vi "SnapImage.vi"(6 "timeout in ms (1000)":i32=1000, 8 "error in (no error)":errorcluster, 11 "Camera":refnum<class "Camera.lvclass">) -> (0 "error out":errorcluster, 2 "buffer":i32=-1, 3 "Camera out":refnum<class "Camera.lvclass">)   [LabVIEW 2015, in "Camera.lvclass"]
doc: "---------------------------------------------------------------\nJKI State Machine Objects™\nhttp://jki.net/state-machine-objects/\nCopyright (C) 2005-2015, JKI <info@jki.net>\nALL RIGHTS RESERVEDJKI State Machine Objects (SMO) 1.0.0.4\nJKI - JKI\nCopyright (c) 2015, JKI"
uses:
  Camera.lvclass
  Camera.lvclass/Camera.ctl
panel:
  # "For instructions on how to use the JKI State Machine Objects, examples and video tutorials, visit:\nhttp://jki.net/state-machine-objects/\n\nJKI State Machine Objects™\nhttp://jki.net/state-machine-objects/\nCopyright (C) 2005-2015, JKI <info@jki.net>\nALL RIGHTS RESERVED"
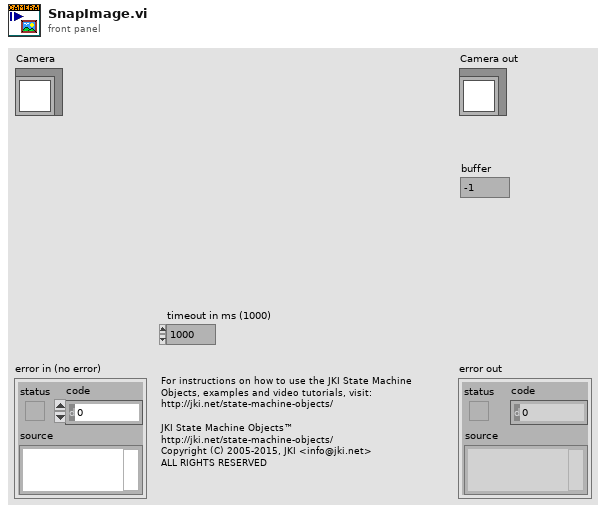
[diagram p1: front panel]
types:
  T1 = typedef "Camera.lvclass/PrivateData--Ref.ctl" = refnum<data-value>
  T2 = typedef "Camera.lvclass/PrivateData--Cluster.ctl" = cluster{"Public Events":T3, "Protected Events":T4, "Private Events":T5, "Dependencies":T6}
  T3 = typedef "Camera.lvclass/PublicEvents--Cluster.ctl" = cluster{"NewImage":refnum<user-event>, "ImageSaved":refnum<user-event>}
  T4 = typedef "Camera.lvclass/ProtectedEvents--Cluster.ctl" = cluster{"placeholder":refnum<user-event>}
  T5 = typedef "Camera.lvclass/PrivateEvents--Cluster.ctl" = cluster{"Snap Image":refnum<user-event>, "Save Image":refnum<user-event>, "Get Image":refnum<user-event>}
  T6 = typedef "Camera.Simulated.lvclass/Dependencies--Cluster.ctl" = cluster{"CircularBuffer.ImageData":refnum<class "CircularBuffer.ImageData.lvclass">}
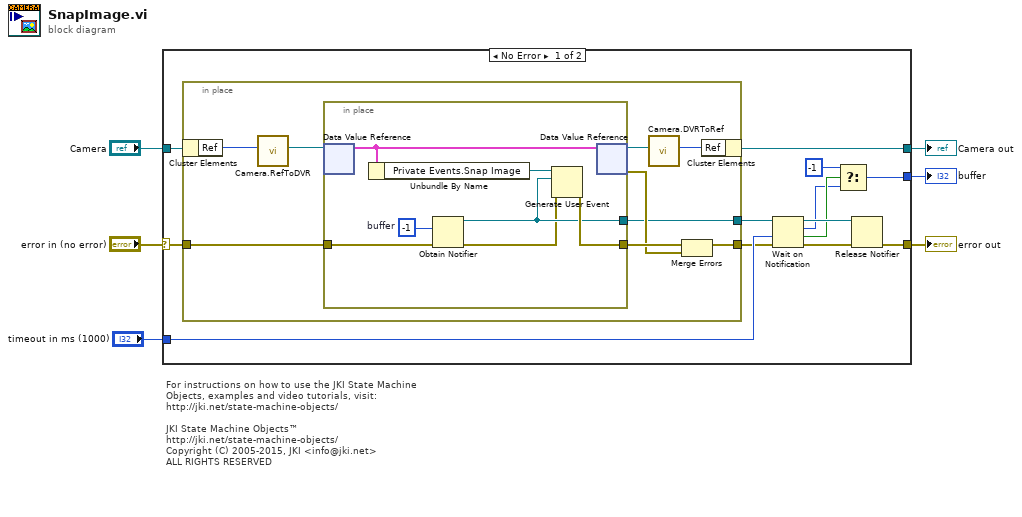
[diagram p0: block diagram]
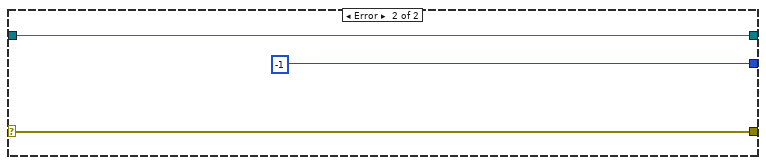
[diagram p2: hidden frame]
diagram:
  # "For instructions on how to use the JKI State Machine Objects, examples and video tutorials, visit:\nhttp://jki.net/state-machine-objects/\n\nJKI State Machine Objects™\nhttp://jki.net/state-machine-objects/\nCopyright (C) 2005-2015, JKI <info@jki.net>\nALL RIGHTS RESERVED"
  n1 = case shown="No Error" "error in (no error)" {
    selector: "error in (no error)" -> [w17 w38]
    tunnel: [w12 w38] -> w5
    tunnel: [w18 w37] -> w6
    tunnel: "Camera" -> [w19 w37]
    tunnel: "timeout in ms (1000)" -> [w15 _]
    tunnel: [w7 -1 ("t")] -> w1
    frame No Error {
      n2 = in-place {
        in-place-border: w17 -> [w28]
        in-place-border: [w25] -> w11
        in-place-border: [w20] -> w16
        n3 = in-place-cluster #1(w19) -> ("Ref"=w24:u32)
        n4 = call "Camera.RefToDVR.vi"("Ref"=w24) -> ("Ref"=w22:T1)  [unwired: 10 in]
        n5 = in-place {
          in-place-border: w28 -> [w30]
          in-place-border: [w33] -> w27
          in-place-border: [w31] -> w20
          w32 = -1  # buffer
          n6 = in-place-dvr #2(w22) -> (w35:T2)  [unwired: 1 out]
          n7 = Unbundle By Name(w35) -> ("Private Events.Snap Image"=w34:refnum<user-event>)
          n8 = Obtain Notifier(notification data type=w32, error in (no error)=w30) -> (notifier out=w31:refnum<notifier>, error out=w29:errorcluster)  [unwired: 2 in, 1 out]
          n9 = Generate User Event(user event=w34, event data cluster=w31, error in=w29) -> (error out=w33:errorcluster)  [unwired: 1 in, 1 out]
          n10 = in-place-dvr #2(w35) -> (w23:T1, w26:errorcluster)
        }
        n11 = call "Camera.DVRToRef.vi"("Ref"=w23) -> ("Ref"=w21:u32)  [unwired: 10 in]
        n12 = Merge Errors(w27, w26) -> (w25:errorcluster)
        n13 = in-place-cluster #1("Ref"=w21) -> (w18:refnum<class "Camera.lvclass">)
      }
      n14 = Wait on Notification(notifier=w16, timeout in ms (-1)=w15, error in (no error)=w11) -> (notifier out=w14:refnum<notifier>, notification=w8:i32, timed out?=w10:bool, error out=w13:errorcluster)  [unwired: 1 in]
      n15 = Select(t=-1, s=w10, f=w8) -> (s? t:f=w7:i32)
      n16 = Release Notifier(notifier=w14, error in (no error)=w13) -> (error out=w12:errorcluster)  [unwired: 1 in, 2 out]
    }
    frame Error {
    }
  }
  "error out" <- w5
  "Camera out" <- w6
  "buffer" <- w1
